vi "setMargins.vi"(7 "Margins":T1, 11 "String in":string) -> (2 "command":string, 3 "String out":string)   [LabVIEW 2012]
uses:
  margins.ctl
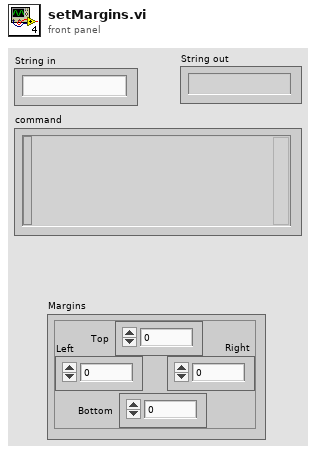
[diagram p1: front panel]
types:
  T1 = typedef "margins.ctl" = cluster{"Top":dbl, "Bottom":dbl, "Left":dbl, "Right":dbl}
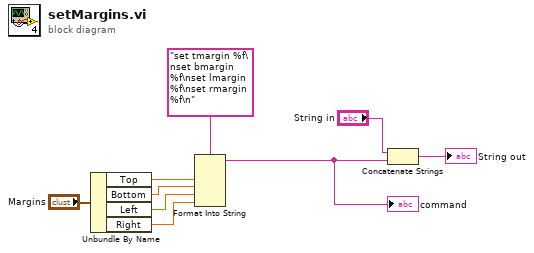
[diagram p0: block diagram]
diagram:
  n1 = Unbundle By Name("Margins") -> ("Top"=w4:dbl, "Bottom"=w3:dbl, "Left"=w2:dbl, "Right"=w1:dbl)
  n2 = Format Into String(format string="set tmargin %f\nset bmargin %f\nset lmargin %f\nset rmargin %f\n", w4, w3, w2, w1) -> (resulting string=w6:string)  [unwired: 2 in, 1 out]
  "command" <- w6
  n3 = Concatenate Strings("String in", w6) -> (→"String out":string)
